vi "Create Frame.vi"(10 "Payload":string, 11 "OpCode":T2) -> (3 "Message Frame":T1)   [LabVIEW 2020, in "Stream-Websocket.lvlib" / "WebsocketStream.lvclass"]
uses:
  WebsocketStream.lvclass
  WebsocketStream.lvclass/WebsocketStream.ctl
  OpCode.ctl
  Stream-Websocket.lvlib
  Message Frame.ctl
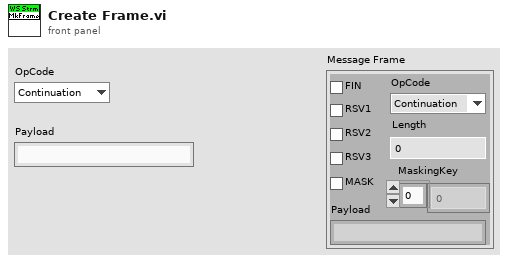
[diagram p1: front panel]
types:
  T1 = typedef "Stream-Websocket.lvlib/Message Frame.ctl" = cluster{"FIN":bool, "RSV1":bool, "RSV2":bool, "RSV3":bool, "MASK":bool, "OpCode":T2, "Length":u64, "MaskingKey":u8[], "Payload":string}
  T2 = typedef "Stream-Websocket.lvlib/OpCode.ctl" = enum8{"Continuation", "Text", "Binary", "Reserved3", "Reserved4", "Reserved5", "Reserved6", "Reserved7", "Close", "Ping", "Pong", "ReservedB", "ReservedC", "ReservedD", "ReservedE", "ReservedF"}
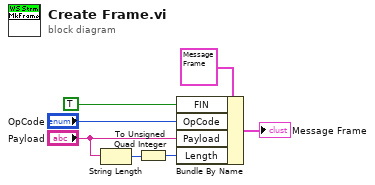
[diagram p0: block diagram]
diagram:
  n1 = String Length(string="Payload") -> (length=w2:i32)
  n2 = To Unsigned Quad Integer(1:w2) -> (0:w1:u64)
  n3 = Bundle By Name(cluster=T1 {"FIN"=FALSE, "RSV1"=FALSE, "RSV2"=FALSE, "RSV3"=FALSE, "MASK"=FALSE, "OpCode"=enum."Continuation", "Length"=0, "MaskingKey"=[], "Payload"=""} ("Message Frame"), "FIN"=TRUE, "OpCode"="OpCode", "Payload"="Payload", "Length"=w1) -> (→"Message Frame":T1)
